vi "Check for valid meid.vi"(8 "error in (no error)":errorcluster, 11 "MEID":string) -> (0 "error out":errorcluster, 3 "Valid MEID":bool)   [LabVIEW 2013]
panel:
  out "sum":i32
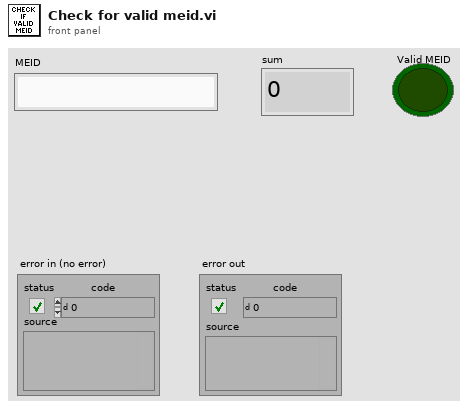
[diagram p1: front panel]
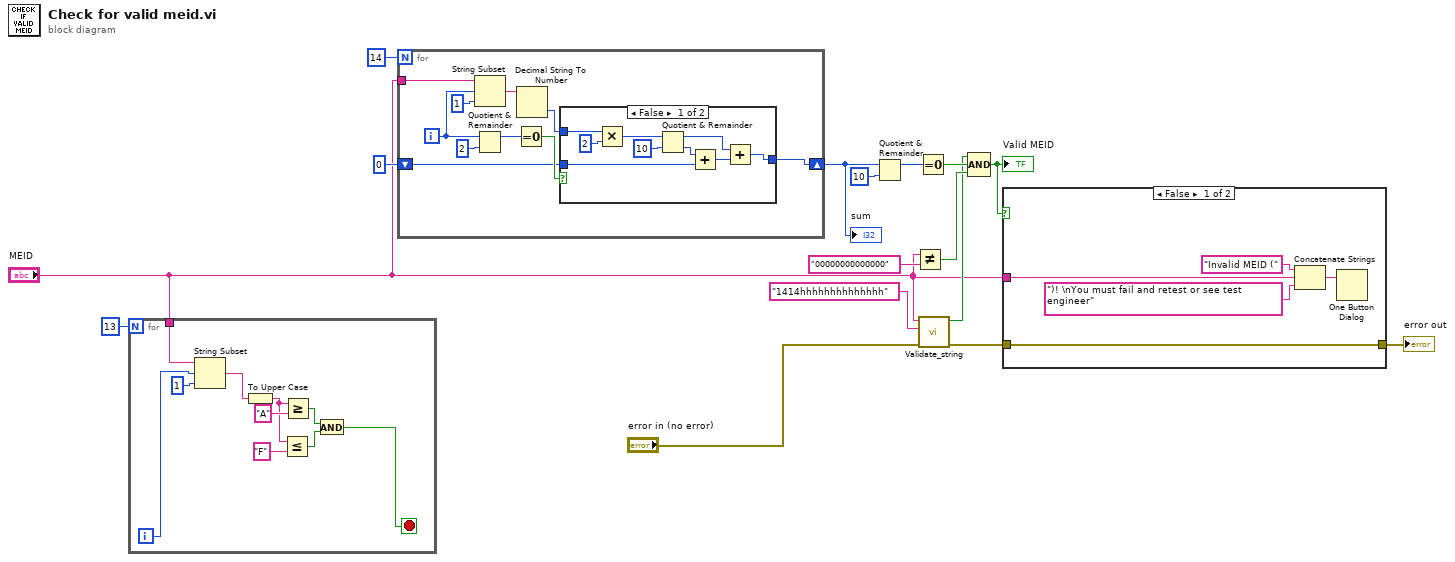
[diagram p0: block diagram]
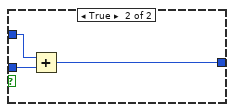
[diagram p3: hidden frame]
diagram:
  n1 = for {
    N: 13 -> [_]
    tunnel: "MEID" -> [w25]
    i -> [w24]
    stop <- w17 stop-if-true
    n2 = String Subset(string=w25, offset (0)=w24, length (rest)=1 ("length (rest)")) -> (substring=w23:string)
    n3 = To Upper Case(1:w23) -> (0:w21:string)
    n4 = Less Or Equal?(x=w21, y="F") -> (x <= y?=w18:bool)
    n5 = Greater Or Equal?(x=w21, y="A") -> (x >= y?=w19:bool)
    n6 = And(x=w19, y=w18) -> (x .and. y?=w17:bool)
  }
  n7 = for {
    N: 14 -> [_]
    tunnel: "MEID" -> [w36]
    shift-right: [w27] -> w14
    shift-left: 0 -> [w28]
    i -> [w34]
    n8 = String Subset(string=w36, offset (0)=w34, length (rest)=1 ("length (rest)")) -> (substring=w30:string)
    n9 = Quotient & Remainder(x=w34, y=2) -> (x-y*floor(x/y)=w32:i32)  [unwired: 1 out]
    n10 = Equal To 0?(x=w32) -> (x = 0?=w31:bool)
    n11 = Decimal String To Number(string=w30) -> (number=w29:i32)  [unwired: 2 in, 1 out]
    n12 = case shown="False" w31 {
      tunnel: w29 -> [w45 w48]
      tunnel: w28 -> [w40 w47]
      tunnel: [w37 w46] -> w27
      frame False {
        n13 = Multiply(x=w45, y=2) -> (x*y=w43:i32)
        n14 = Quotient & Remainder(x=w43, y=10) -> (x-y*floor(x/y)=w39:i32, floor(x/y)=w41:i32)
        n15 = Add(x=w41, y=w40) -> (x+y=w38:i32)
        n16 = Add(x=w39, y=w38) -> (x+y=w37:i32)
      }
      frame True {
        n17 = Add(x=w48, y=w47) -> (x+y=w46:i32)
      }
    }
  }
  "sum" <- w14
  n18 = Quotient & Remainder(x=w14, y=10) -> (x-y*floor(x/y)=w12:i32)  [unwired: 1 out]
  n19 = Not Equal?(x="MEID", y="00000000000000") -> (x != y?=w10:bool)
  n20 = Equal To 0?(x=w12) -> (x = 0?=w9:bool)
  n21 = call "Validate_string.vi"("error in (no error)"="error in (no error)", "String data format"="1414hhhhhhhhhhhhhh", "String"="MEID") -> ("error out"=w4:errorcluster, "String Valid"=w3:bool)  [unwired: 7 in]
  n22 = Compound Arithmetic op=AND(w3, w9, w10) -> (w8:bool)
  "Valid MEID" <- w8
  n23 = case shown="False" w8 {
    tunnel: [w53 w54] -> w7
    tunnel: w4 -> [w53 w54]
    tunnel: "MEID" -> [w51 _]
    frame False {
      n24 = Concatenate Strings("Invalid MEID (" ("message"), w51, ")! \nYou must fail and retest or see test engineer" ("message")) -> (w49:string)
      n25 = One Button Dialog(message=w49) -> ()  [unwired: 1 in, 1 out]
    }
    frame True {
    }
  }
  "error out" <- w7
